vi "Begin.vi"(8 "error in":errorcluster) -> (0 "error out":errorcluster)   [LabVIEW 2020]
doc: "Called before other user functions, this VI is expected to open initial I/O refnums, load in file data, and do all program initialization. Notice that the <B>error out</B> terminal is simply used for data flow. Wiring it to other structures or subVIs ensures that this VI runs first."
uses:
  <vilib>/Rock Robotics/WPI/DriverStation/WPI_DriverStationRobotMode2.ctl
  <vilib>/Rock Robotics/WPI/Joystick/WPI_JoystickDeviceEnum.ctl
  <vilib>/Rock Robotics/WPI/SafetyOutput/WPI_SafetyOutputConfigMenu.ctl
  Robot Global Data.vi
  <vilib>/Rock Robotics/Network Tables/NT Write String Array.vi
  Color-Sensor-v3-Examples-master/LabVIEW/Color Match/Global 1.vi
  <vilib>/Rock Robotics/WPI/RobotDrive/WPI_RobotDriveOpen2MotorWithExistingMotors.vi
  <vilib>/Rock Robotics/WPI/MotorControl/WPI_MotorControlDeviceRef.ctl
  <vilib>/Rock Robotics/SystemInterfaces/DIO/FPGA_DIOPWMChannel.ctl
  <vilib>/Rock Robotics/WPI/PWM/WPI_PWMDeadband.ctl
  <vilib>/Rock Robotics/WPI/MotorControl/WPI_MotorControlType.ctl
  <vilib>/Rock Robotics/SystemInterfaces/DIO/FPGA_DIOChannel.ctl
panel:
  out "error out shooter":errorcluster
  out "Shooter Motor Group":T1={"DeviceStatus"={"status"=FALSE, "code"=0, "source"=""}, "Type"=enum."CAN", "PWM"={"PWM Channel"=enum."Invalid", "DeadBand"={"Name"="", "maxPositivePwm"=0, "minPositivePwm"=0, "centerPwm"=0, "maxNegativePwm"=0, "minNegativePwm"=0, "angularRange"=0}}, "CAN"={"Device Number"=7, "SetOutput VI Ref"=variant, "GetOutput VI Ref"=variant, "Enable VI Ref"=variant, "Disable VI Ref"=variant, "Data"=variant}, "Invert"=FALSE, "DIO PWM"={"PWM \"Enable\" Channel"=enum."Invalid", "DIOChannel"=enum."Invalid", "PWM Rate"=0.0}}
  out "error out angle":errorcluster
  out "Angle Motor Group":T1={"DeviceStatus"={"status"=FALSE, "code"=0, "source"=""}, "Type"=enum."CAN", "PWM"={"PWM Channel"=enum."Invalid", "DeadBand"={"Name"="", "maxPositivePwm"=0, "minPositivePwm"=0, "centerPwm"=0, "maxNegativePwm"=0, "minNegativePwm"=0, "angularRange"=0}}, "CAN"={"Device Number"=7, "SetOutput VI Ref"=variant, "GetOutput VI Ref"=variant, "Enable VI Ref"=variant, "Disable VI Ref"=variant, "Data"=variant}, "Invert"=FALSE, "DIO PWM"={"PWM \"Enable\" Channel"=enum."Invalid", "DIOChannel"=enum."Invalid", "PWM Rate"=0.0}}
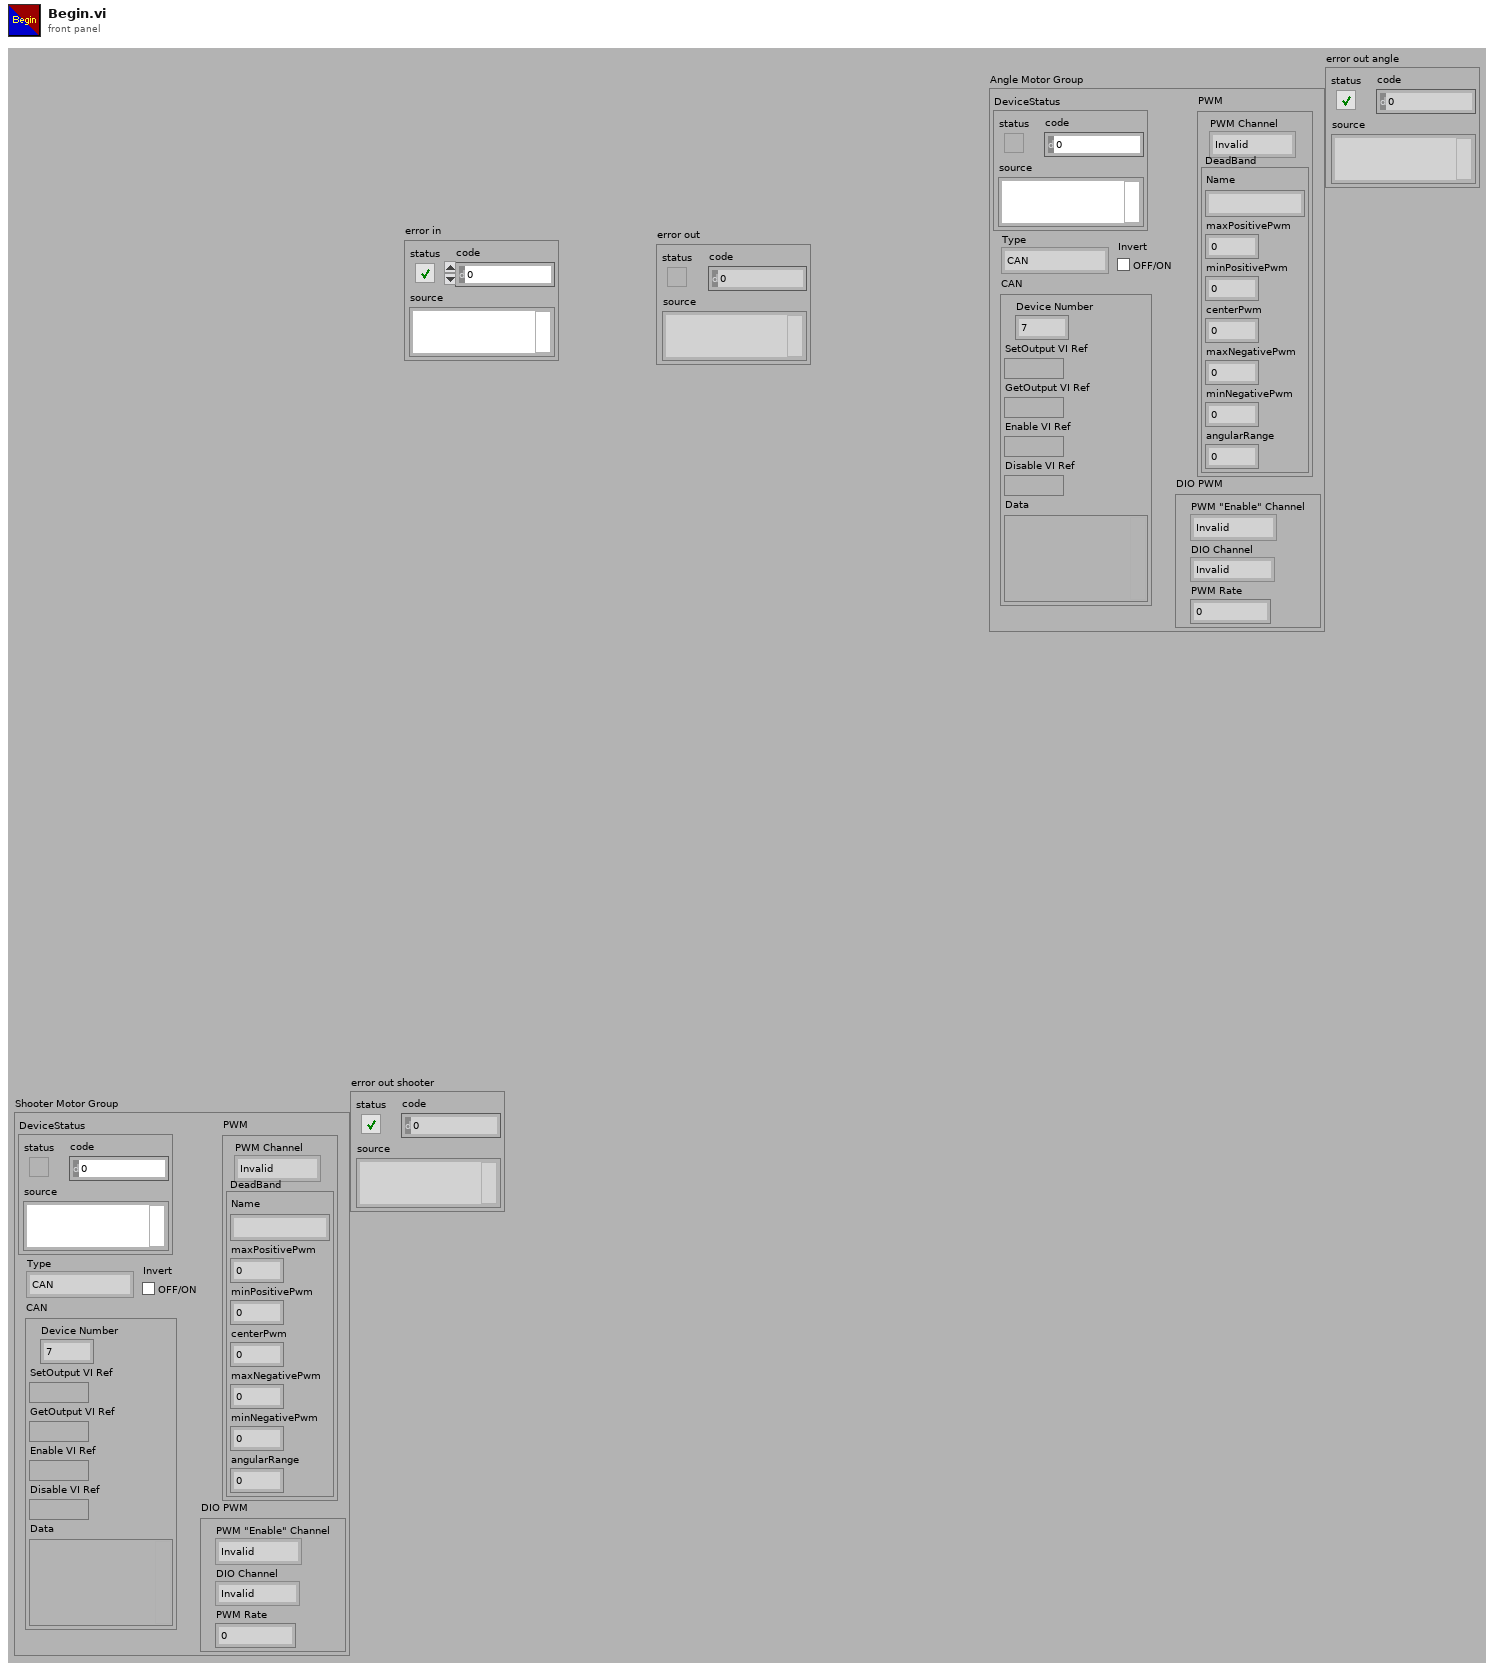
[diagram p1: front panel]
types:
  T1 = typedef "WPI_MotorControlDeviceRef.ctl" = cluster{"DeviceStatus":errorcluster, "Type":T2, "PWM":cluster{"PWM Channel":T3, "DeadBand":T4}, "CAN":cluster{"Device Number":u8, "SetOutput VI Ref":variant, "GetOutput VI Ref":variant, "Enable VI Ref":variant, "Disable VI Ref":variant, "Data":variant}, "Invert":bool, "DIO PWM":cluster{"PWM \"Enable\" Channel":T3, "DIOChannel":T5, "PWM Rate":dbl}}
  T2 = typedef "WPI_MotorControlType.ctl" = enum16{"PWM", "CAN", "DIO PWM"}
  T3 = typedef "FPGA_DIOPWMChannel.ctl" = enum8{"PWM 0", "PWM 1", "PWM 2", "PWM 3", "PWM 4", "PWM 5", "PWM 6", "PWM 7", "PWM 8", "PWM 9", "PWM MXP 0", "PWM MXP 1", "PWM MXP 2", "PWM MXP 3", "PWM MXP 4", "PWM MXP 5", "PWM MXP 6", "PWM MXP 7", "PWM MXP 8", "PWM MXP 9", "Invalid"}
  T4 = typedef "WPI_PWMDeadband.ctl" = cluster{"Name":string, "maxPositivePwm":i32, "minPositivePwm":i32, "centerPwm":i32, "maxNegativePwm":i32, "minNegativePwm":i32, "angularRange":u16}
  T5 = typedef "FPGA_DIOChannel.ctl" = enum8{"DIO 0", "DIO 1", "DIO 2", "DIO 3", "DIO 4", "DIO 5", "DIO 6", "DIO 7", "DIO 8", "DIO 9", "DIO MXP 0", "DIO MXP 1", "DIO MXP 2", "DIO MXP 3", "DIO MXP 4", "DIO MXP 5", "DIO MXP 6", "DIO MXP 7", "DIO MXP 8", "DIO MXP 9", "DIO MXP 10", "DIO MXP 11", "DIO MXP 12", "DIO MXP 13", "DIO MXP 14", "DIO MXP 15", "SPI Port CS1", "SPI Port CS2", "SPI Port CS3", "SPI Port MISO", "SPI Port MOSI", "Invalid"}
  T6 = typedef "WPI_SafetyOutputConfigMenu.ctl" = enum16{"Enable", "Disable"}
  T7 = typedef "WPI_JoystickDeviceEnum.ctl" = enum16{"USB 0", "USB 1", "USB 2", "USB 3", "USB 4", "USB 5"}
  T8 = typedef "WPI_DriverStationRobotMode2.ctl" = enum16{"Autonomous Disabled", "Autonomous Enabled", "Teleop Disabled", "Teleop Enabled", "Disconnected", "Finish", "Test Disabled", "Test Enabled", "Emergency Stopped"}
  T9 = typedef "WPI_EncoderDevRef.ctl" = cluster{"DevStatus":errorcluster, "EncoderIndex":T10, "CounterIndex":T11, "DistancePerCount":dbl, "Decoding Type":T12}
  T10 = typedef "FPGA_EncoderIdx.ctl" = enum8{"Enc 0", "Enc 1", "Enc 2", "Enc 3", "Enc 4", "Enc 5", "Enc 6", "Enc 7", "Invalid"}
  T11 = typedef "FPGA_CounterCtrSystemIndex.ctl" = enum8{"Ctr 0", "Ctr 1", "Ctr 2", "Ctr 3", "Ctr 4", "Ctr 5", "Ctr 6", "Ctr 7", "Invalid"}
  T12 = typedef "WPI_EncoderType.ctl" = enum16{"1x", "2x", "4x"}
  T13 = typedef "WPI_RobotDriveDevRef.ctl" = cluster{"DevStatus":errorcluster, "Motors[]":T1[], "Square Inputs":bool, "Max Output":dbl}
  T14 = typedef "WPI_JoystickDevRef.ctl" = cluster{"Device":T7}
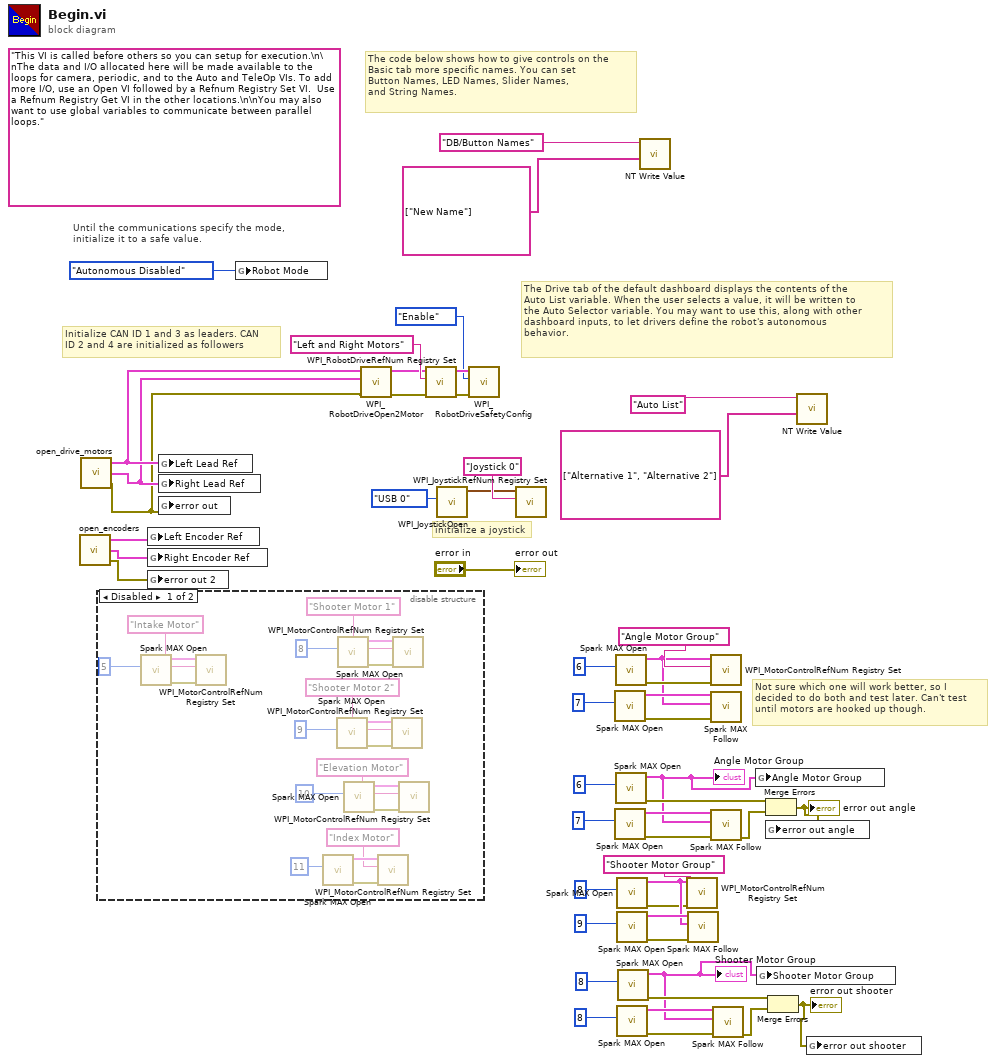
[diagram p0: block diagram]
diagram:
  (unwired) "This VI is called before others so you can setup for execution.\n\nThe data and I/O allocated here will be made available to the loops for camera, periodic, and to the Auto and TeleOp VIs. To add more I/O, use an Open VI followed by a Refnum Registry Set VI.  Use a Refnum Registry Get VI in the other locations.\n\nYou may also want to use global variables to communicate between parallel loops."
  # "Not sure which one will work better, so I\ndecided to do both and test later. Can't test \nuntil motors are hooked up though."
  # "The Drive tab of the default dashboard displays the contents of the\nAuto List variable. When the user selects a value, it will be written to\nthe Auto Selector variable. You may want to use this, along with other\ndashboard inputs, to let drivers define the robot's autonomous\nbehavior."
  # "The code below shows how to give controls on the\nBasic tab more specific names. You can set\nButton Names, LED Names, Slider Names,\nand String Names."
  # "initialize a joystick"
  # "Until the communications specify the mode,\ninitialize it to a safe value."
  # "Initialize CAN ID 1 and 3 as leaders. CAN \nID 2 and 4 are initialized as followers"
  n1 = call "open_encoders.vi"() -> ("error out"=w35:errorcluster, "Right Encoder Ref"=w36:T9, "Left Encoder Ref"=w37:T9)
  n2 = call "open_drive_motors.vi"() -> ("error out"=w32:errorcluster, "Right Lead Ref"=w33:T1, "Left Lead Ref"=w34:T1)
  n3 = disable-structure shown="Disabled" {
    frame Disabled {
      n4 = call <vilib>:"Spark MAX Open.vi"("Device Number"=u8 5) -> ("error out"=w70:errorcluster, "MotorControlDeviceRef"=w69:T1)  [unwired: 9 in]
      n5 = call <vilib>:"WPI_MotorControlRefNum Registry Set.vi"("error in (no error)"=w70, "refnum name"="Intake Motor", "MotorControlDevRef"=w69) -> ()  [unwired: 7 in, 2 out]
      n6 = call <vilib>:"Spark MAX Open.vi"("Device Number"=u8 11) -> ("error out"=w62:errorcluster, "MotorControlDeviceRef"=w61:T1)  [unwired: 9 in]
      n7 = call <vilib>:"Spark MAX Open.vi"("Device Number"=u8 9) -> ("error out"=w54:errorcluster, "MotorControlDeviceRef"=w53:T1)  [unwired: 9 in]
      n8 = call <vilib>:"Spark MAX Open.vi"("Device Number"=u8 8) -> ("error out"=w58:errorcluster, "MotorControlDeviceRef"=w57:T1)  [unwired: 9 in]
      n9 = call <vilib>:"Spark MAX Open.vi"("Device Number"=u8 10) -> ("error out"=w67:errorcluster, "MotorControlDeviceRef"=w66:T1)  [unwired: 9 in]
      n10 = call <vilib>:"WPI_MotorControlRefNum Registry Set.vi"("error in (no error)"=w62, "refnum name"="Index Motor", "MotorControlDevRef"=w61) -> ()  [unwired: 7 in, 2 out]
      n11 = call <vilib>:"WPI_MotorControlRefNum Registry Set.vi"("error in (no error)"=w54, "refnum name"="Shooter Motor 2", "MotorControlDevRef"=w53) -> ()  [unwired: 7 in, 2 out]
      n12 = call <vilib>:"WPI_MotorControlRefNum Registry Set.vi"("error in (no error)"=w58, "refnum name"="Shooter Motor 1", "MotorControlDevRef"=w57) -> ()  [unwired: 7 in, 2 out]
      n13 = call <vilib>:"WPI_MotorControlRefNum Registry Set.vi"("error in (no error)"=w67, "refnum name"="Elevation Motor", "MotorControlDevRef"=w66) -> ()  [unwired: 7 in, 2 out]
    }
    frame Enabled {
    }
  }
  n14 = global write "Global 1.vi" "Left Encoder Ref"(w37) -> ()
  n15 = global write "Global 1.vi" "Right Encoder Ref"(w36) -> ()
  n16 = global write "Global 1.vi" "error out 2"(w35) -> ()
  n17 = global write "Global 1.vi" "Left Lead Ref"(w34) -> ()
  n18 = global write "Global 1.vi" "Right Lead Ref"(w33) -> ()
  n19 = global write "Global 1.vi" "error out"(w32) -> ()
  n20 = global write "Robot Global Data.vi" "Robot Mode"(WPI_DriverStationRobotMode2."Autonomous Disabled" ("Robot Mode")) -> ()
  n21 = call-poly <vilib>:"WPI_RobotDriveOpen2Motor.vi"("error in (no error)"=w32, "Right Motor Dev Ref"=w33, "Left Motor Dev Ref"=w34) -> ("error out"=w40:errorcluster, "RobotDriveDevRef"=w38:T13)  [unwired: 7 in]
  n22 = call <vilib>:"WPI_RobotDriveRefNum Registry Set.vi"("error in (no error)"=w40, "refnum name"="Left and Right Motors", "RobotDriveDevRef"=w38) -> ("error out"=w43:errorcluster, "RobotDriveDevRef"=w42:T13)  [unwired: 7 in]
  n23 = call <vilib>:"WPI_JoystickOpen.vi"("JoystickDevice"=WPI_JoystickDeviceEnum."USB 0") -> ("JoystickDevRef"=w49:T14)  [unwired: 10 in]
  n24 = call <vilib>:"WPI_RobotDriveSafetyConfig.vi"("error in (no error)"=w43, "mode"=WPI_SafetyOutputConfigMenu."Enable", "RobotDriveDevRef"=w42) -> ()  [unwired: 7 in, 2 out]
  n25 = call <vilib>:"WPI_JoystickRefNum Registry Set.vi"("refnum name"="Joystick 0", "JoystickDevRef"=w49) -> ()  [unwired: 8 in, 2 out]
  n26 = call <vilib>:"Spark MAX Open.vi"("Device Number"=u8 7) -> ("error out"=w25:errorcluster, "MotorControlDeviceRef"=w26:T1)  [unwired: 9 in]
  n27 = call <vilib>:"Spark MAX Open.vi"("Device Number"=u8 7) -> ("error out"=w20:errorcluster, "MotorControlDeviceRef"=w21:T1)  [unwired: 9 in]
  n28 = call <vilib>:"Spark MAX Open.vi"("Device Number"=u8 6) -> ("error out"=w28:errorcluster, "MotorControlDeviceRef"=w24:T1)  [unwired: 9 in]
  n29 = call <vilib>:"Spark MAX Open.vi"("Device Number"=u8 6) -> ("error out"=w18:errorcluster, "MotorControlDeviceRef"=w17:T1)  [unwired: 9 in]
  "Angle Motor Group" <- w17
  n30 = call <vilib>:"Spark MAX Open.vi"("Device Number"=u8 8) -> ("error out"=w10:errorcluster, "MotorControlDeviceRef"=w11:T1)  [unwired: 9 in]
  n31 = call <vilib>:"Spark MAX Open.vi"("Device Number"=u8 9) -> ("error out"=w12:errorcluster, "MotorControlDeviceRef"=w13:T1)  [unwired: 9 in]
  n32 = call <vilib>:"Spark MAX Open.vi"("Device Number"=u8 8) -> ("error out"=w5:errorcluster, "MotorControlDeviceRef"=w6:T1)  [unwired: 9 in]
  n33 = call <vilib>:"Spark MAX Open.vi"("Device Number"=u8 8) -> ("error out"=w3:errorcluster, "MotorControlDeviceRef"=w1:T1)  [unwired: 9 in]
  "Shooter Motor Group" <- w1
  n34 = call-poly <vilib>:"NT Write Value.vi"("String Array"=string[] ["New Name"], "Name"="DB/Button Names") -> ()  [unwired: 9 in, 1 out]
  n35 = call <vilib>:"WPI_MotorControlRefNum Registry Set.vi"("error in (no error)"=w10, "refnum name"="Shooter Motor Group", "MotorControlDevRef"=w11) -> ()  [unwired: 7 in, 2 out]
  n36 = call <vilib>:"Spark MAX Follow.vi"("error in (no error)"=w12, "Master Controller"=w11, "MotorControlDeviceRef"=w13) -> ()  [unwired: 7 in, 2 out]
  n37 = call <vilib>:"WPI_MotorControlRefNum Registry Set.vi"("error in (no error)"=w28, "refnum name"="Angle Motor Group", "MotorControlDevRef"=w24) -> ()  [unwired: 7 in, 2 out]
  n38 = call <vilib>:"Spark MAX Follow.vi"("error in (no error)"=w25, "Master Controller"=w24, "MotorControlDeviceRef"=w26) -> ()  [unwired: 7 in, 2 out]
  n39 = call <vilib>:"Spark MAX Follow.vi"("error in (no error)"=w20, "Master Controller"=w17, "MotorControlDeviceRef"=w21) -> ("error out"=w19:errorcluster)  [unwired: 7 in, 1 out]
  n40 = call <vilib>:"Spark MAX Follow.vi"("error in (no error)"=w5, "Master Controller"=w1, "MotorControlDeviceRef"=w6) -> ("error out"=w4:errorcluster)  [unwired: 7 in, 1 out]
  n41 = global write "Global 1.vi" "Angle Motor Group"(w17) -> ()
  n42 = global write "Global 1.vi" "Shooter Motor Group"(w1) -> ()
  n43 = Merge Errors(w18, w19) -> (w16:errorcluster)
  "error out angle" <- w16
  n44 = global write "Global 1.vi" "error out angle"(w16) -> ()
  n45 = Merge Errors(w3, w4) -> (w2:errorcluster)
  "error out shooter" <- w2
  n46 = call-poly <vilib>:"NT Write Value.vi"("String Array"=string[] ["Alternative 1", "Alternative 2"], "Name"="Auto List") -> ()  [unwired: 9 in, 1 out]
  n47 = global write "Global 1.vi" "error out shooter"(w2) -> ()
  "error out" <- "error in"
